vi "Motor-Maker-Square RD.vi"() -> ()   [LabVIEW 2014]
panel:
  in  "Liga desliga":bool
  out "N Quadrados":i32
  in  "Lado Volta":dbl
  in  "Base Volta":dbl
  in  "Lado ida":dbl
  in  "Base X ida":dbl
  out "Motor Y\nLigado Volta":bool=TRUE
  out "Motor X\nLigado Volta":bool=TRUE
  out "Motor Y\nLigado ida":bool=TRUE
  out "Motor X\nLigado ida":bool=TRUE
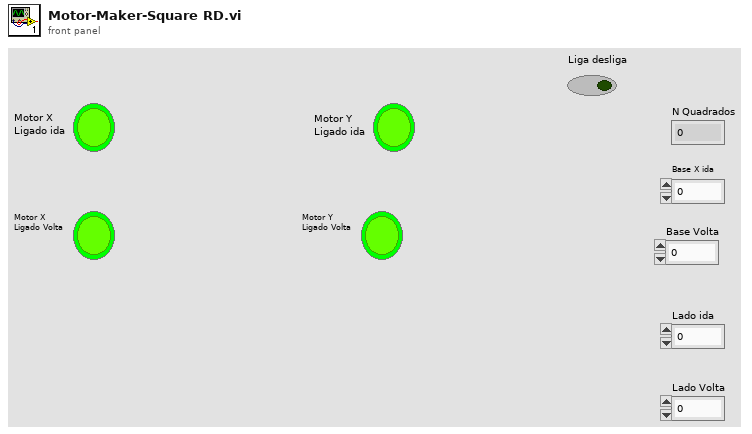
[diagram p1: front panel]
types:
  T1 = enum16{"Motor X ida", "Motor Y ida", "Motor X Volta", "Motor Y Volta"}
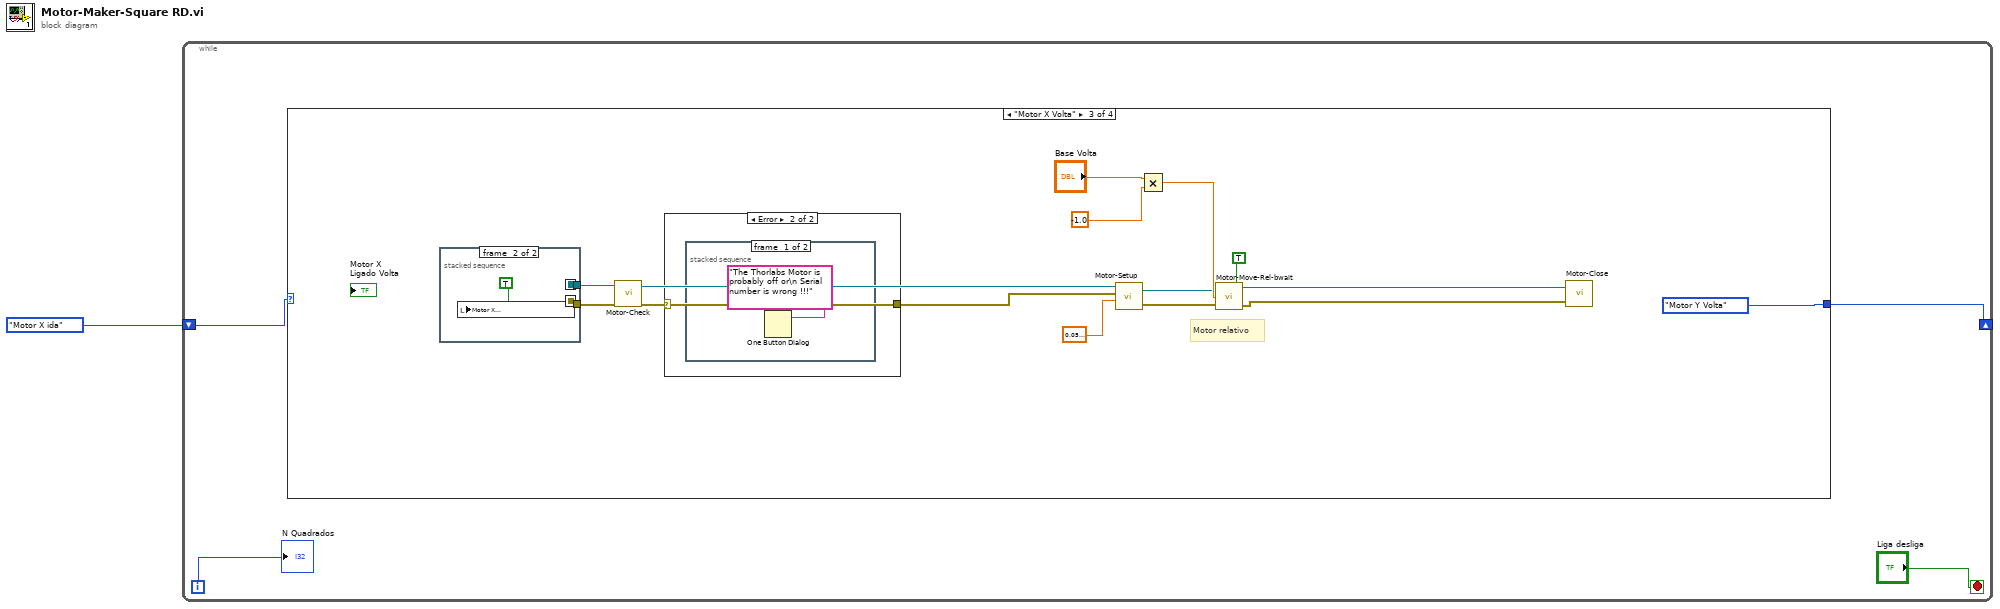
[diagram p0: block diagram]
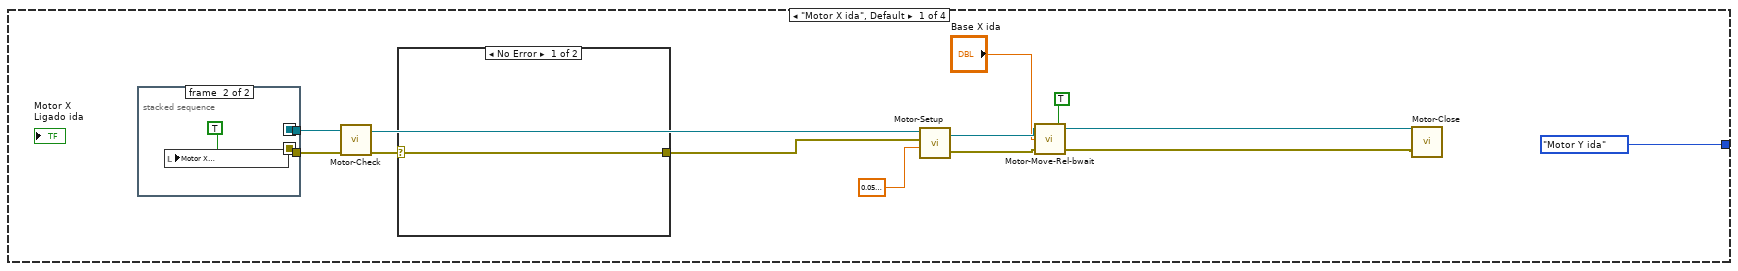
[diagram p2: hidden frame]
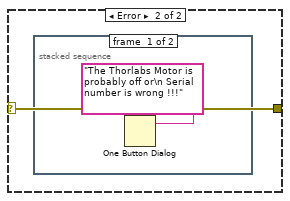
[diagram p3: hidden frame]
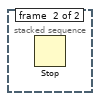
[diagram p4: hidden frame]
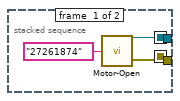
[diagram p5: hidden frame]
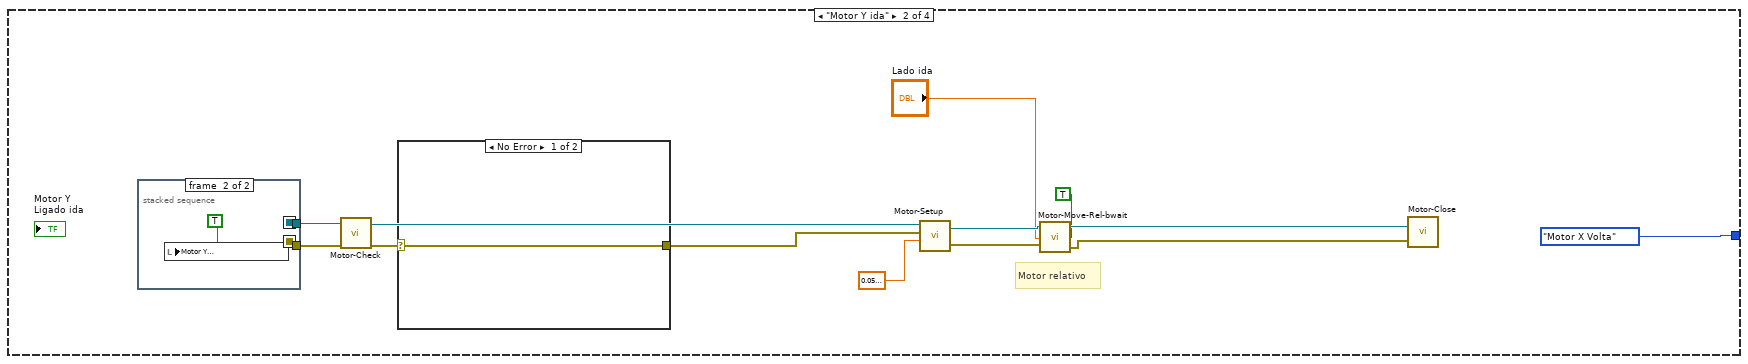
[diagram p6: hidden frame]
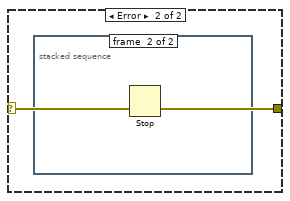
[diagram p7: hidden frame]
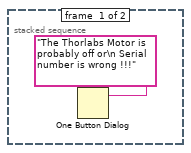
[diagram p8: hidden frame]
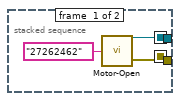
[diagram p9: hidden frame]
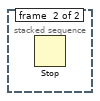
[diagram p11: hidden frame]
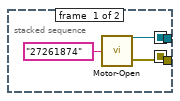
[diagram p12: hidden frame]
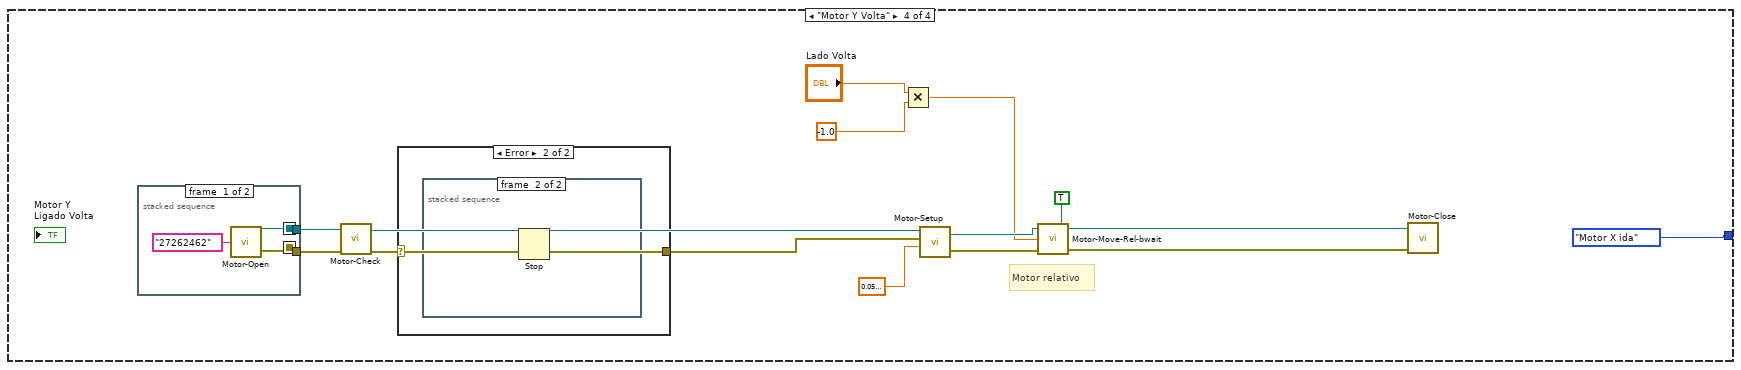
[diagram p13: hidden frame]
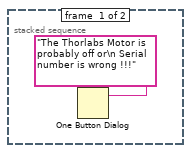
[diagram p15: hidden frame]
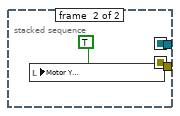
[diagram p16: hidden frame]
diagram:
  n1 = while {
    shift-right: [w4] -> _
    shift-left: T1."Motor X ida" -> [w5]
    i -> [w3]
    stop <- "Liga desliga" stop-if-true
    n2 = case shown="\"Motor X Volta\"" w5 {
      tunnel: [T1."Motor Y ida" T1."Motor X Volta" T1."Motor Y Volta" T1."Motor X ida"] -> w4
      frame "Motor X ida", Default {
        n3 = stacked-sequence {
          seq-local: [w24 _] -> [_ w27]
          seq-local: [w23 _] -> [_ w26]
          tunnel: [_ w27] -> w18
          tunnel: [_ w26] -> w17
          frame #0 {
            n4 = call "Motor-Open.vi"("S/N Motor"="27261874") -> ("MG17Motor 2"=w24:refnum<k7>, "error out"=w23:errorcluster)
          }
          frame #1 {
            n5 = local write "Motor X\nLigado ida"(TRUE ("Motor3\nLigado")) -> ()
          }
        }
        n6 = call "Motor-Check.vi"("error in (no error)"=w17, "Automation Refnum in"=w18) -> ("error out"=w16:errorcluster, "Automation Refnum out"=w15:refnum<k7>)  [unwired: 8 in]
        n7 = case shown="No Error" w16 {
          selector: w16 -> [w19 w20]
          tunnel: [w19 w20] -> w14
          frame No Error {
          }
          frame Error {
            n8 = stacked-sequence {
              frame #0 {
                n9 = One Button Dialog(message="The Thorlabs Motor is probably off or\n Serial number is wrong !!!") -> ()  [unwired: 1 in, 1 out]
              }
              frame #1 {
                n10 = Stop() -> ()  [unwired: 1 in]
              }
            }
          }
        }
        n11 = call "Motor-Setup.vi"("Velocidade"=sgl 0.05, "error"=w14, "MG17Motor A"=w15) -> ("error out"=w7:errorcluster, "MG17Motor out"=w8:refnum<k7>)  [unwired: 1 in]
        n12 = call "Motor-Move-Rel-bwait.vi"("bWait"=TRUE, "error"=w7, "Posição"="Base X ida", "MG17Motor A"=w8) -> ("error out"=w10:errorcluster, "MG17Motor out"=w9:refnum<k7>)
        n13 = call "Motor-Close.vi"("error out"=w10, "MG17Motor 3"=w9) -> ()  [unwired: 1 in]
      }
      frame "Motor Y ida" {
        # "Motor relativo"
        n14 = stacked-sequence {
          seq-local: [w46 _] -> [_ w49]
          seq-local: [w45 _] -> [_ w48]
          tunnel: [_ w49] -> w40
          tunnel: [_ w48] -> w39
          frame #0 {
            n15 = call "Motor-Open.vi"("S/N Motor"="27262462") -> ("MG17Motor 2"=w46:refnum<k7>, "error out"=w45:errorcluster)
          }
          frame #1 {
            n16 = local write "Motor Y\nLigado ida"(TRUE ("Motor3\nLigado")) -> ()
          }
        }
        n17 = call "Motor-Check.vi"("error in (no error)"=w39, "Automation Refnum in"=w40) -> ("error out"=w38:errorcluster, "Automation Refnum out"=w37:refnum<k7>)  [unwired: 8 in]
        n18 = case shown="No Error" w38 {
          selector: w38 -> [w41 w42]
          tunnel: [w41 w42] -> w36
          frame No Error {
          }
          frame Error {
            n19 = stacked-sequence {
              frame #0 {
                n20 = One Button Dialog(message="The Thorlabs Motor is probably off or\n Serial number is wrong !!!") -> ()  [unwired: 1 in, 1 out]
              }
              frame #1 {
                n21 = Stop() -> ()  [unwired: 1 in]
              }
            }
          }
        }
        n22 = call "Motor-Setup.vi"("Velocidade"=sgl 0.05, "error"=w36, "MG17Motor A"=w37) -> ("error out"=w32:errorcluster, "MG17Motor out"=w33:refnum<k7>)  [unwired: 1 in]
        n23 = call "Motor-Move-Rel-bwait.vi"("bWait"=TRUE, "error"=w32, "Posição"="Lado ida", "MG17Motor A"=w33) -> ("error out"=w31:errorcluster, "MG17Motor out"=w29:refnum<k7>)
        n24 = call "Motor-Close.vi"("error out"=w31, "MG17Motor 3"=w29) -> ()  [unwired: 1 in]
      }
      frame "Motor X Volta" {
        # "Motor relativo"
        n25 = stacked-sequence {
          seq-local: [w70 _] -> [_ w73]
          seq-local: [w69 _] -> [_ w72]
          tunnel: [_ w73] -> w64
          tunnel: [_ w72] -> w63
          frame #0 {
            n26 = call "Motor-Open.vi"("S/N Motor"="27261874") -> ("MG17Motor 2"=w70:refnum<k7>, "error out"=w69:errorcluster)
          }
          frame #1 {
            n27 = local write "Motor X\nLigado Volta"(TRUE ("Motor3\nLigado")) -> ()
          }
        }
        n28 = call "Motor-Check.vi"("error in (no error)"=w63, "Automation Refnum in"=w64) -> ("error out"=w62:errorcluster, "Automation Refnum out"=w61:refnum<k7>)  [unwired: 8 in]
        n29 = case shown="Error" w62 {
          selector: w62 -> [w65 w66]
          tunnel: [w65 w66] -> w60
          frame No Error {
          }
          frame Error {
            n30 = stacked-sequence {
              frame #0 {
                n31 = One Button Dialog(message="The Thorlabs Motor is probably off or\n Serial number is wrong !!!") -> ()  [unwired: 1 in, 1 out]
              }
              frame #1 {
                n32 = Stop() -> ()  [unwired: 1 in]
              }
            }
          }
        }
        n33 = call "Motor-Setup.vi"("Velocidade"=sgl 0.05, "error"=w60, "MG17Motor A"=w61) -> ("error out"=w51:errorcluster, "MG17Motor out"=w52:refnum<k7>)  [unwired: 1 in]
        n34 = Multiply(x="Base Volta", y=-1.0) -> (x*y=w53:dbl)
        n35 = call "Motor-Move-Rel-bwait.vi"("bWait"=TRUE, "error"=w51, "Posição"=w53, "MG17Motor A"=w52) -> ("error out"=w54:errorcluster, "MG17Motor out"=w55:refnum<k7>)
        n36 = call "Motor-Close.vi"("error out"=w54, "MG17Motor 3"=w55) -> ()  [unwired: 1 in]
      }
      frame "Motor Y Volta" {
        # "Motor relativo"
        n37 = stacked-sequence {
          seq-local: [w94 _] -> [_ w97]
          seq-local: [w93 _] -> [_ w96]
          tunnel: [_ w97] -> w88
          tunnel: [_ w96] -> w87
          frame #0 {
            n38 = call "Motor-Open.vi"("S/N Motor"="27262462") -> ("MG17Motor 2"=w94:refnum<k7>, "error out"=w93:errorcluster)
          }
          frame #1 {
            n39 = local write "Motor Y\nLigado Volta"(TRUE ("Motor3\nLigado")) -> ()
          }
        }
        n40 = call "Motor-Check.vi"("error in (no error)"=w87, "Automation Refnum in"=w88) -> ("error out"=w86:errorcluster, "Automation Refnum out"=w85:refnum<k7>)  [unwired: 8 in]
        n41 = case shown="Error" w86 {
          selector: w86 -> [w89 w90]
          tunnel: [w89 w90] -> w84
          frame No Error {
          }
          frame Error {
            n42 = stacked-sequence {
              frame #0 {
                n43 = One Button Dialog(message="The Thorlabs Motor is probably off or\n Serial number is wrong !!!") -> ()  [unwired: 1 in, 1 out]
              }
              frame #1 {
                n44 = Stop() -> ()  [unwired: 1 in]
              }
            }
          }
        }
        n45 = Multiply(x="Lado Volta", y=-1.0) -> (x*y=w75:dbl)
        n46 = call "Motor-Setup.vi"("Velocidade"=sgl 0.05, "error"=w84, "MG17Motor A"=w85) -> ("error out"=w78:errorcluster, "MG17Motor out"=w77:refnum<k7>)  [unwired: 1 in]
        n47 = call "Motor-Move-Rel-bwait.vi"("bWait"=TRUE, "error"=w78, "Posição"=w75, "MG17Motor A"=w77) -> ("error out"=w79:errorcluster, "MG17Motor out"=w80:refnum<k7>)
        n48 = call "Motor-Close.vi"("error out"=w79, "MG17Motor 3"=w80) -> ()  [unwired: 1 in]
      }
    }
    "N Quadrados" <- w3
  }
